vi "refence_test.vi"() -> ()   [LabVIEW 2013]
panel:
  out "数值":i32
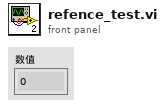
[diagram p1: front panel]
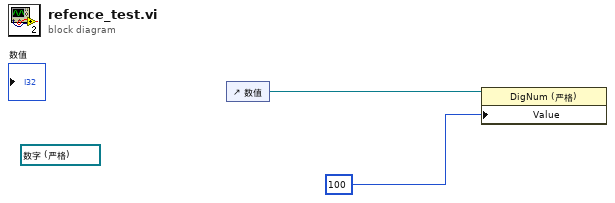
[diagram p0: block diagram]
diagram:
  (unwired) refnum<vi> refnum ("数值")
  n1 = control-ref of="数值"() -> (w2:refnum<vi>)
  n2 = property class="DigNum (严格)"(reference=w2, "Value"=100 ("值")) -> ()  [unwired: 1 in, 2 out]
